vi "Basis VI.vi"() -> ()   [LabVIEW 2013]
uses:
  <vilib>/userdefined/High Color/nirio_resource_hc.ctl
  cRIO_FPGA_COMMUNICATION/TYPES/TYPE Station Index.ctl
  <vilib>/ImagingLab/Kawasaki Robotics Library/typedefs/KwRL-cartesian.ctl
  cRIO_FPGA_COMMUNICATION/GLOBALS/cRIO_FPGA_COMMUNICATION Global.vi
  <vilib>/ImagingLab/Kawasaki Robotics Library/sub/poly/kwrl-motion-move-move_linear(pos).vi
  cRIO_FPGA_COMMUNICATION/cRIO_FPGA_COMMUNICATION.lvlib
  <vilib>/ImagingLab/Kawasaki Robotics Library/KawasakiRoboticsLibrary.lvlib
panel:
  in  "STOP":bool
  in  "WIEDERANFAHRT":bool
  in  "HALT":bool
  in  "START":bool
  in  "demontage oder ausschuss":bool
  in  "Zylinder Festhalten":bool
  in  "Zylinder Bolzen":bool
  in  "value 2":bool
  in  "value":bool
  in  "position 2":T1 {"S" format="%.4g"; "T" format="%.4g"; "A" format="%.4g"; "O" format="%.4g"; "Z" format="%.4g"; "Y" format="%.4g"; "X" format="%.4g"}
  out "MA":bool
  out "Zählerwert 2":u16
  in  "gewünschter Zählerwert 2":u16
  out "Rucksetzen":bool
  in  "Fahr":bool
  in  "Schleichfahrt":bool
  in  "LF":bool
  in  "RF":bool
  out "Impulsgeber":bool
  out "RA":bool
  out "LA":bool
  in  "Band/Station Index (Position im Prozess)":T2
  out "Station":bool[](array[boolean])
  out "Band":bool[](array[boolean])
  in  "Station":bool[](array[boolean])=[FALSE, FALSE, FALSE, FALSE, FALSE, FALSE, FALSE, FALSE]
  in  "Band":bool[](array[boolean])=[FALSE, FALSE, FALSE, FALSE, FALSE, FALSE, FALSE, FALSE]
  in  "Ressourcenname":T3 caption="RIO Device"
  in  "Stopp":bool
  # "Basis VI für allgemeine Stationen"
  # "Senden"
  # "Empfangen"
  # "0      1      2     3     4     5     6     7"
  # "0      1      2     3     4     5     6     7"
  # "Empfangen"
  # "Senden"
  # "0      1      2     3     4     5     6     7"
  # "0      1      2     3     4     5     6     7"
  # "Sensoren"
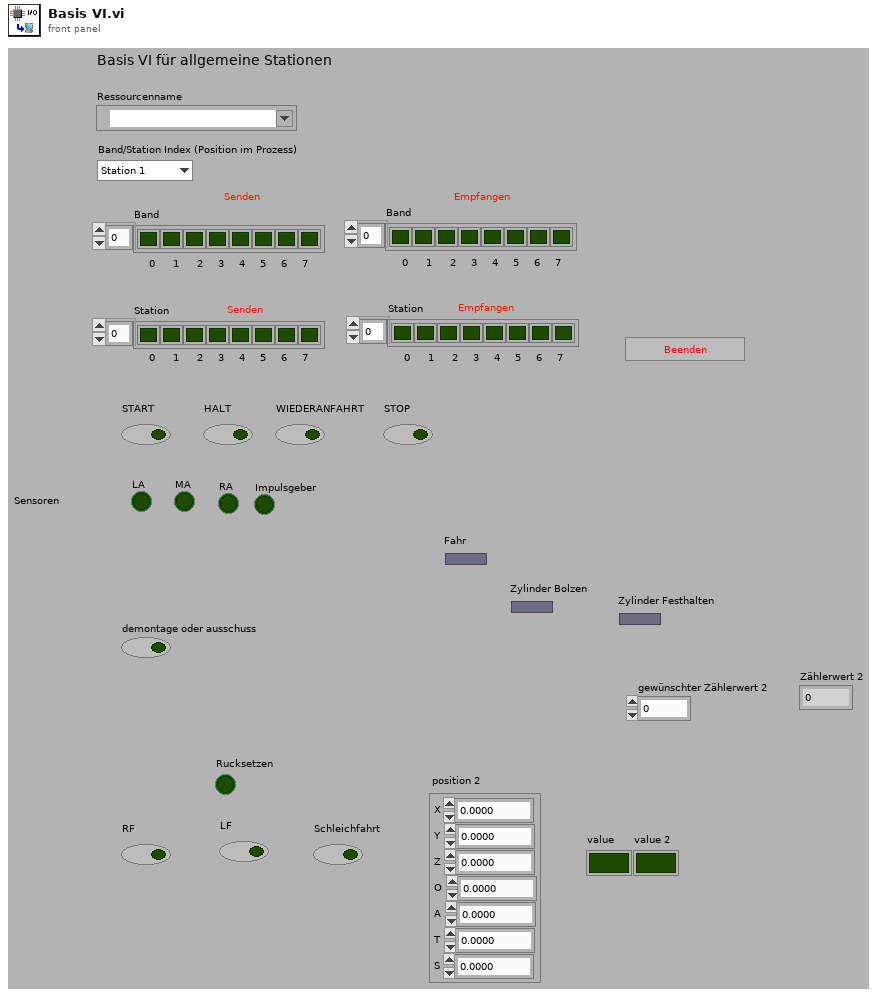
[diagram p1: front panel]
types:
  T1 = typedef "KawasakiRoboticsLibrary.lvlib/kwrl-cartesian.ctl" = cluster{"X":dbl, "Y":dbl, "Z":dbl, "O":dbl, "A":dbl, "T":dbl, "S":dbl}
  T2 = typedef "cRIO_FPGA_COMMUNICATION.lvlib/TYPE Station Index.ctl" = enum16{"Station 1", "Station 2", "Station 3", "Station 4", "Station 5", "Station 6", "Station 7", "Station 8", "Station 9", "Station 10", "Station 11", "Station 12", "Station 13", "Station 14", "Station 15", "Station 16", "Station 17", "Station 18", "Station 19", "Station 20"}
  T3 = typedef "nirio_resource_hc.ctl" = tag
  T4 = typedef "KawasakiRoboticsLibrary.lvlib/KwRL-cartesian.ctl" = cluster{"X":dbl, "Y":dbl, "Z":dbl, "O":dbl, "A":dbl, "T":dbl, "S":dbl}
  T5 = enum16{"Bereit", "Linksfahrt", "Rechtsfahrt 1", "Rechts- und Schleichfahrt", "Stop", "abholen", "demontagepos", "ausschuss", "deckel", "bolzen", "grundkorper", "rechtsfahrt2", "ende"}
  T6 = typedef "TYPE Zählerkonfiguration.ctl" = cluster{"Station/Band":enum16{"Station", "Band"}, "Bitstelle":enum16{"Bit 0", "Bit 1", "Bit 2", "Bit 3", "Bit 4", "Bit 5", "Bit 6", "Bit 7"}, "Zählrichtung":enum16{"Hochzählen", "Runterzählen"}}
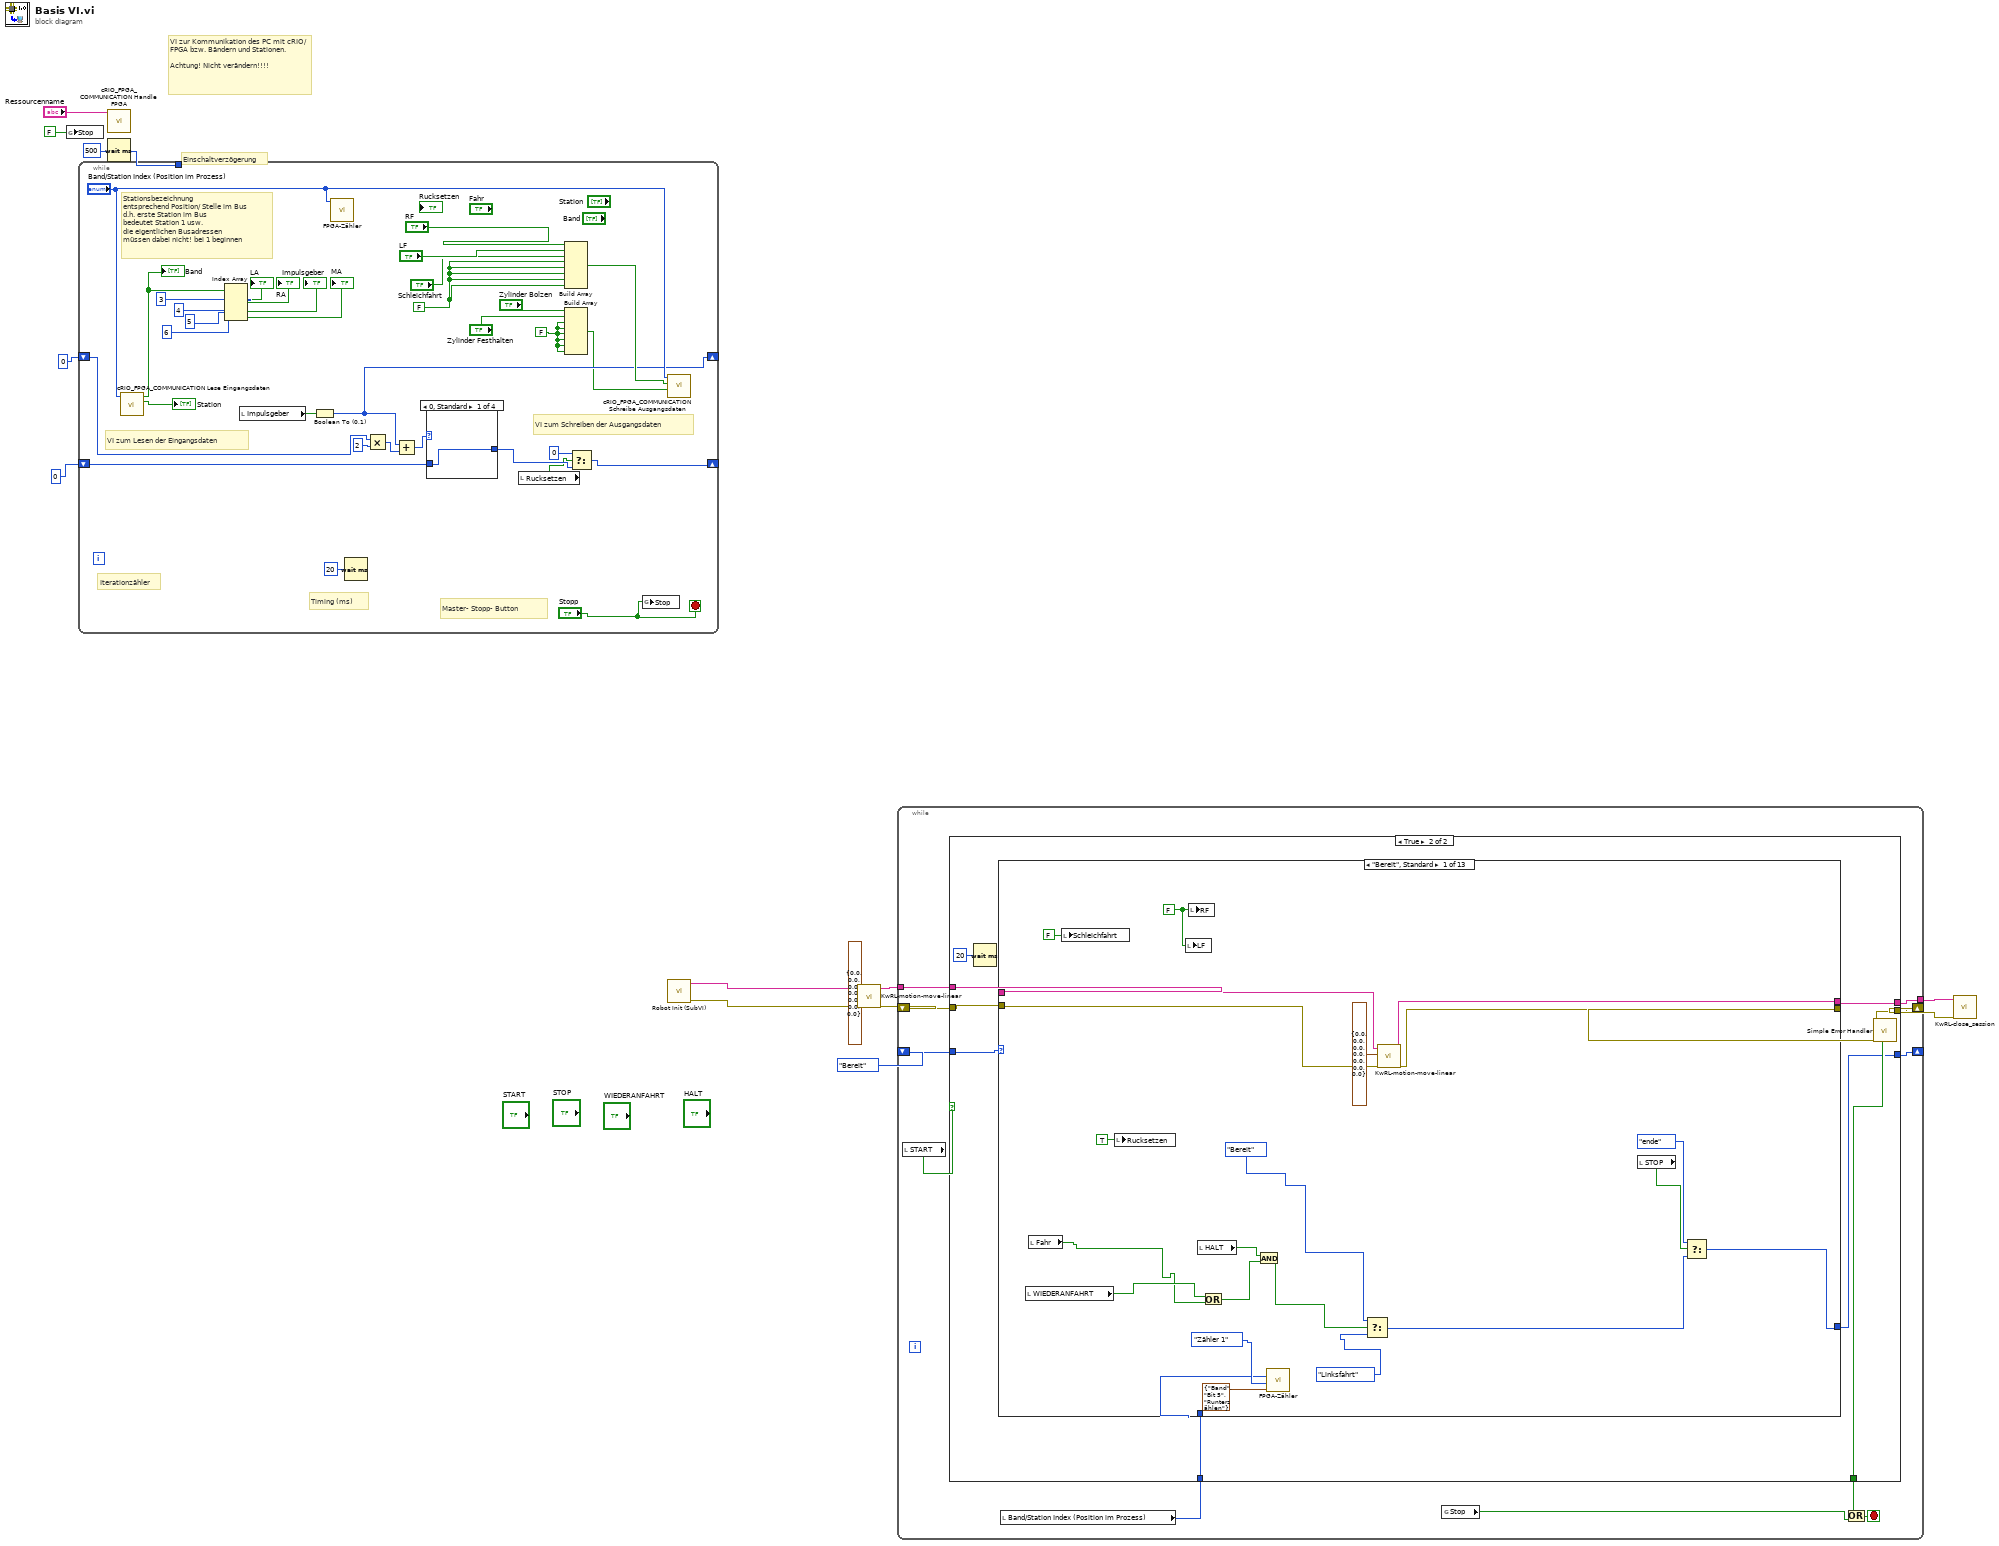
[diagram p0: block diagram]
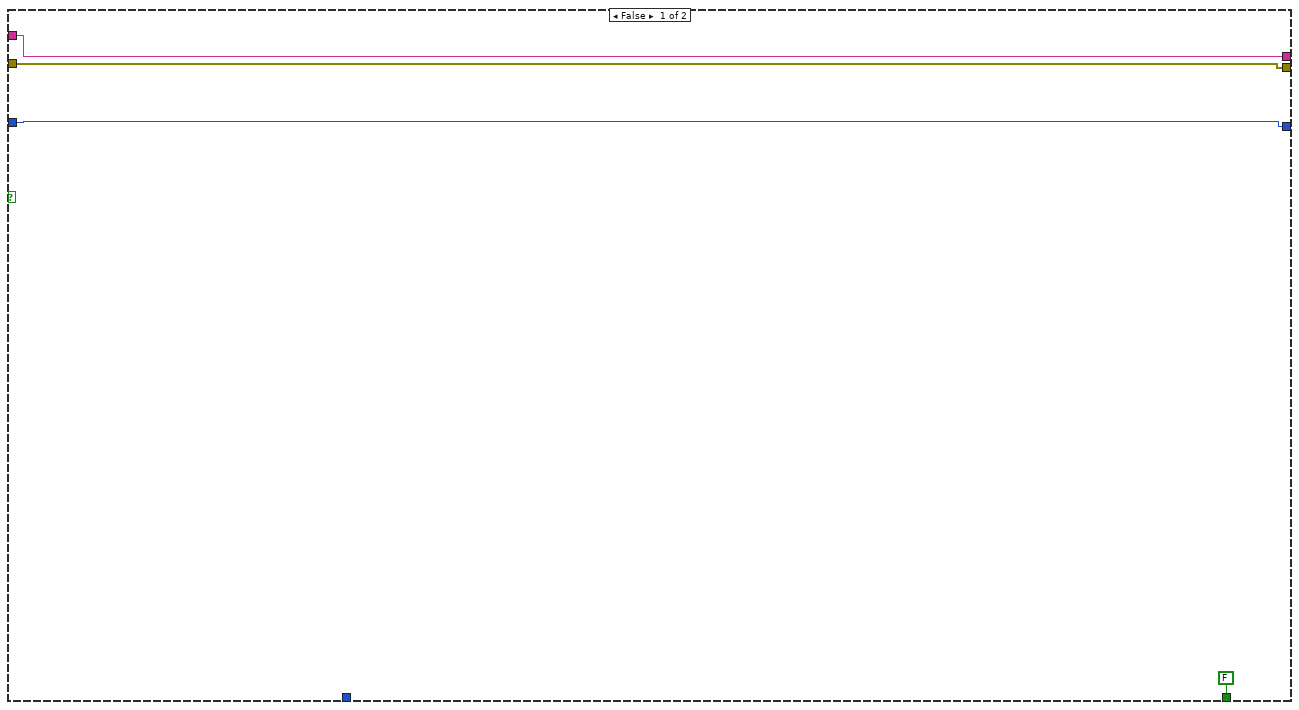
[diagram p2: hidden frame]
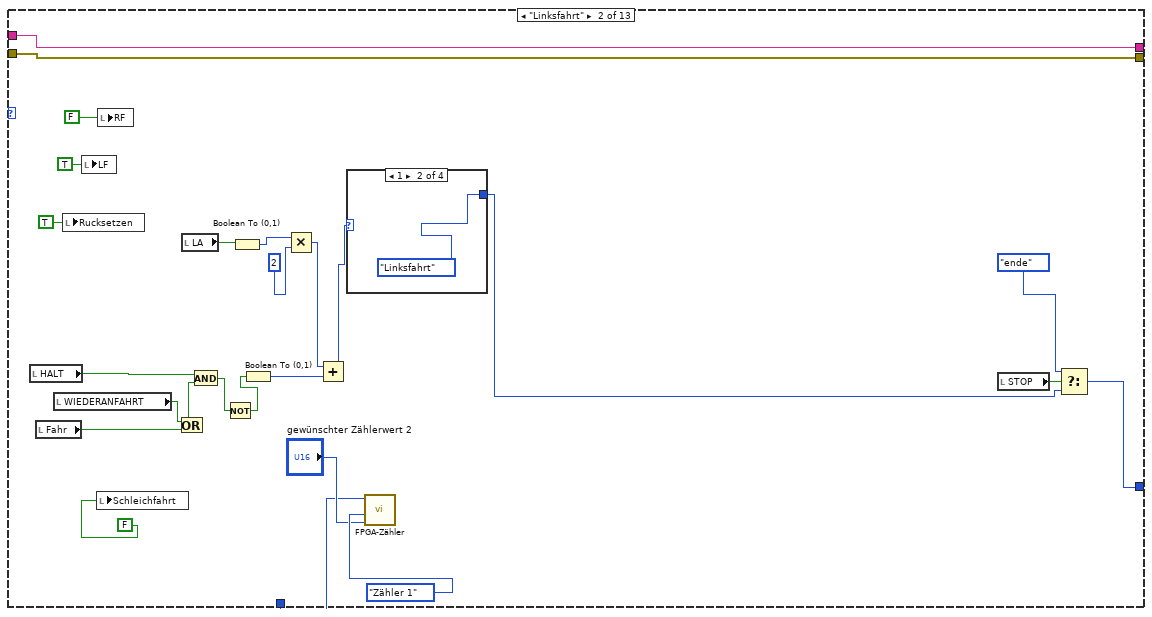
[diagram p3: hidden frame]
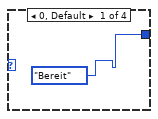
[diagram p4: hidden frame]
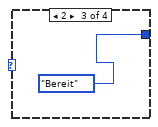
[diagram p5: hidden frame]
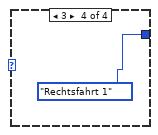
[diagram p6: hidden frame]
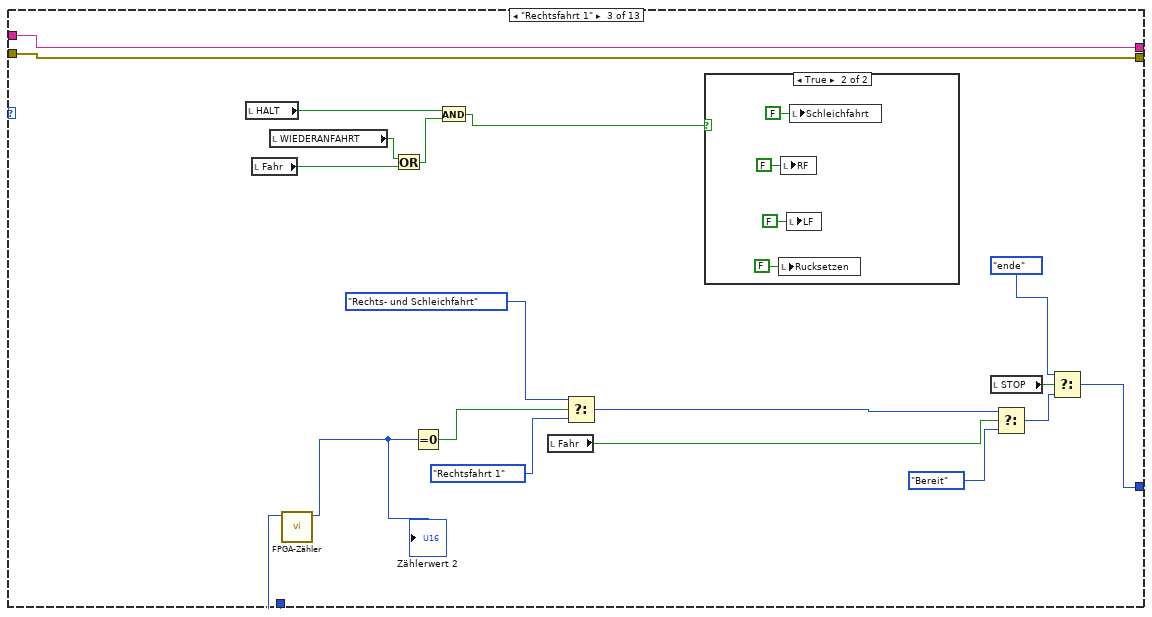
[diagram p7: hidden frame]
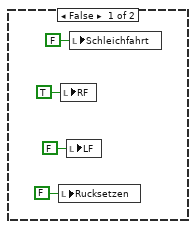
[diagram p8: hidden frame]
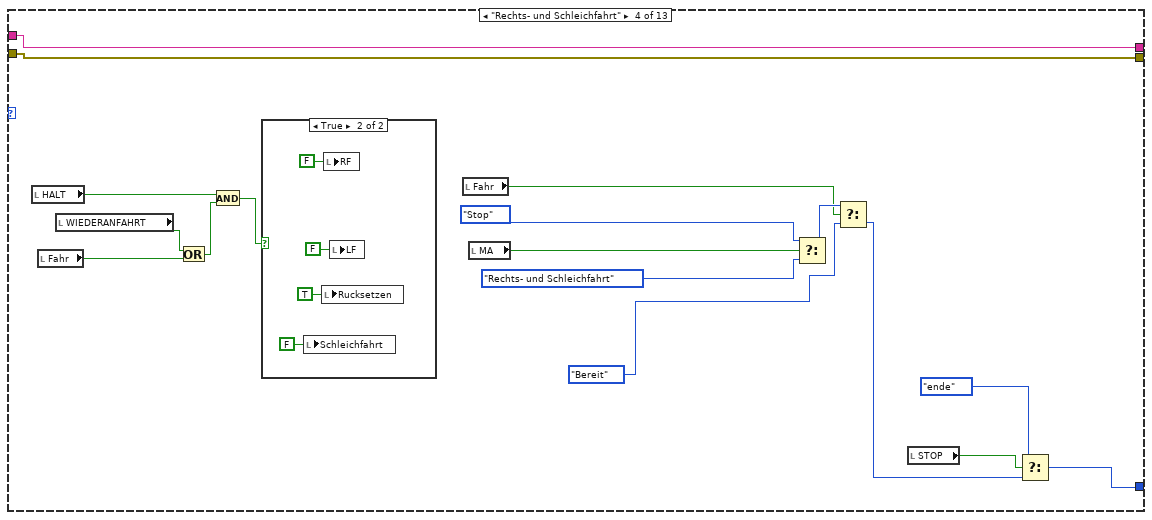
[diagram p9: hidden frame]
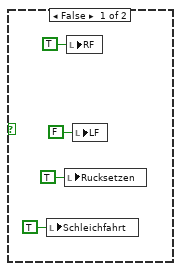
[diagram p10: hidden frame]
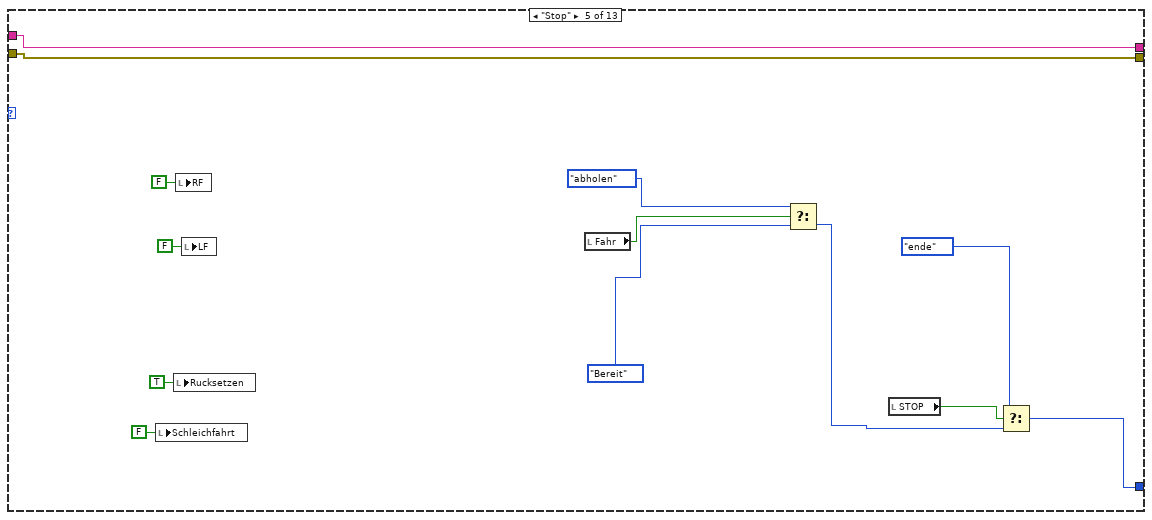
[diagram p11: hidden frame]
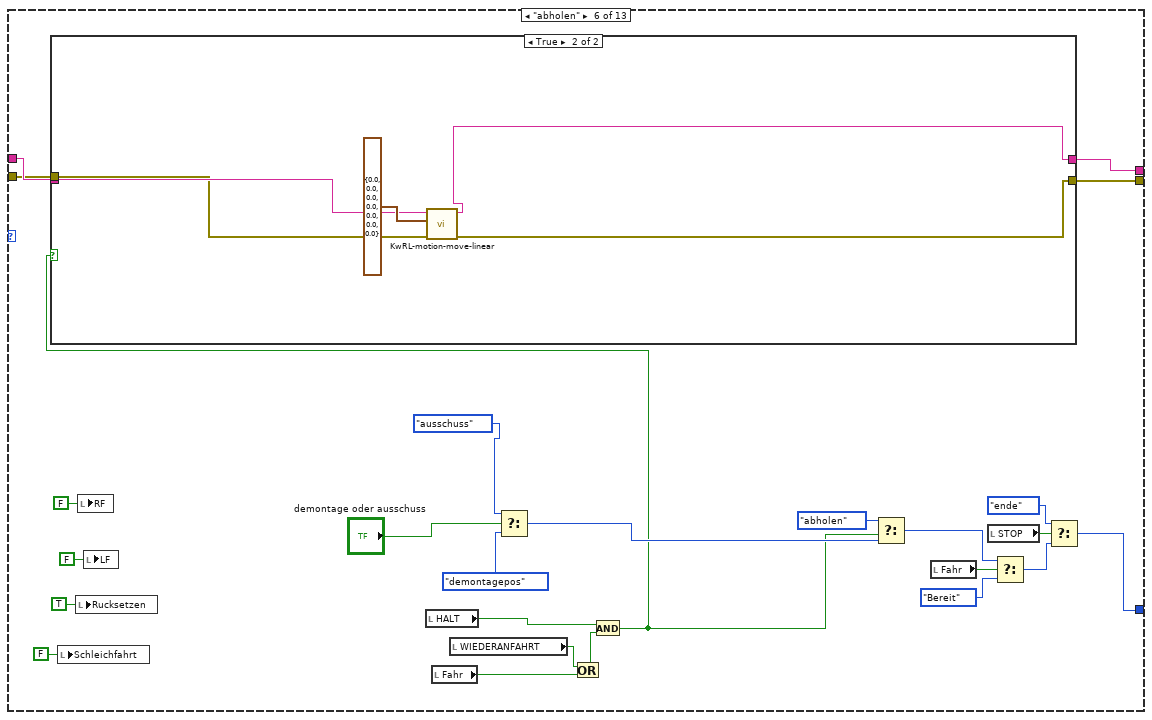
[diagram p12: hidden frame]
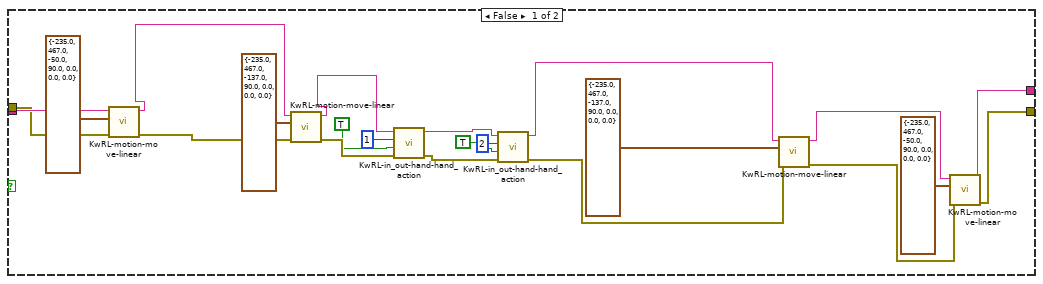
[diagram p13: hidden frame]
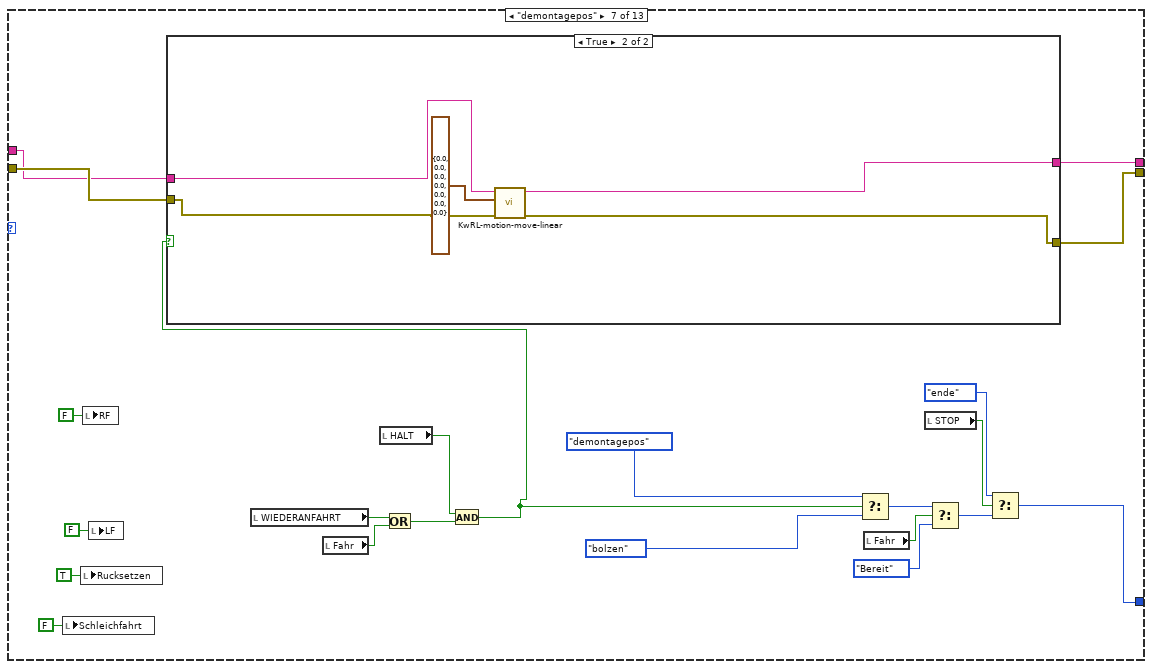
[diagram p14: hidden frame]
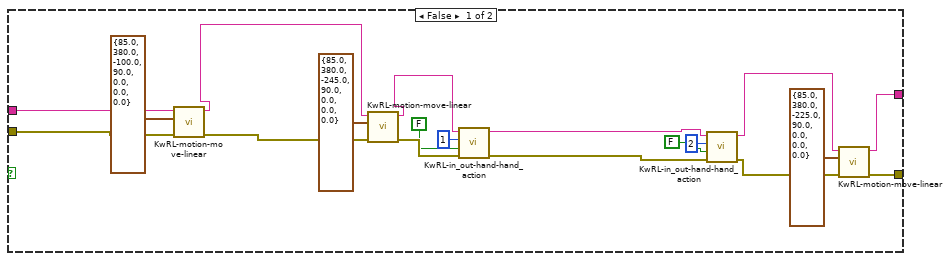
[diagram p15: hidden frame]
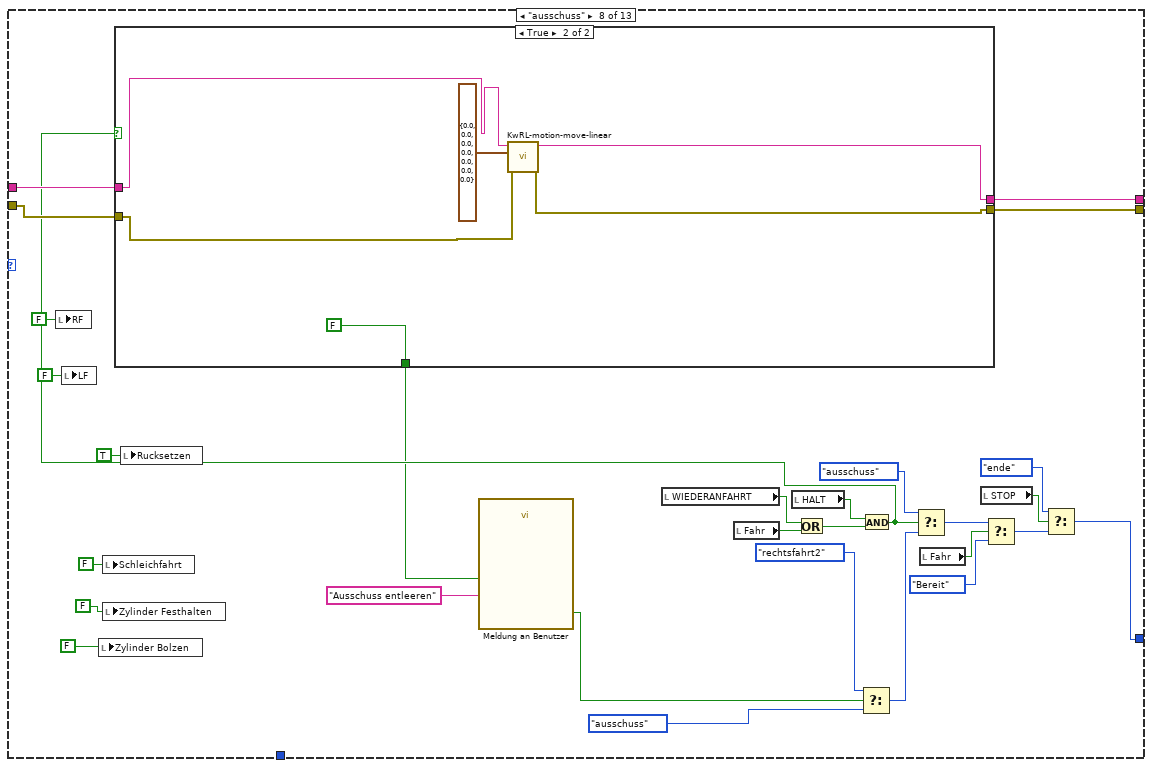
[diagram p16: hidden frame]
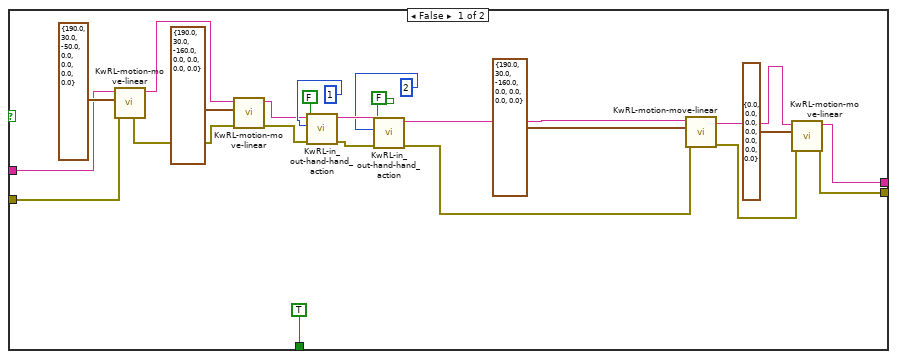
[diagram p17: hidden frame]
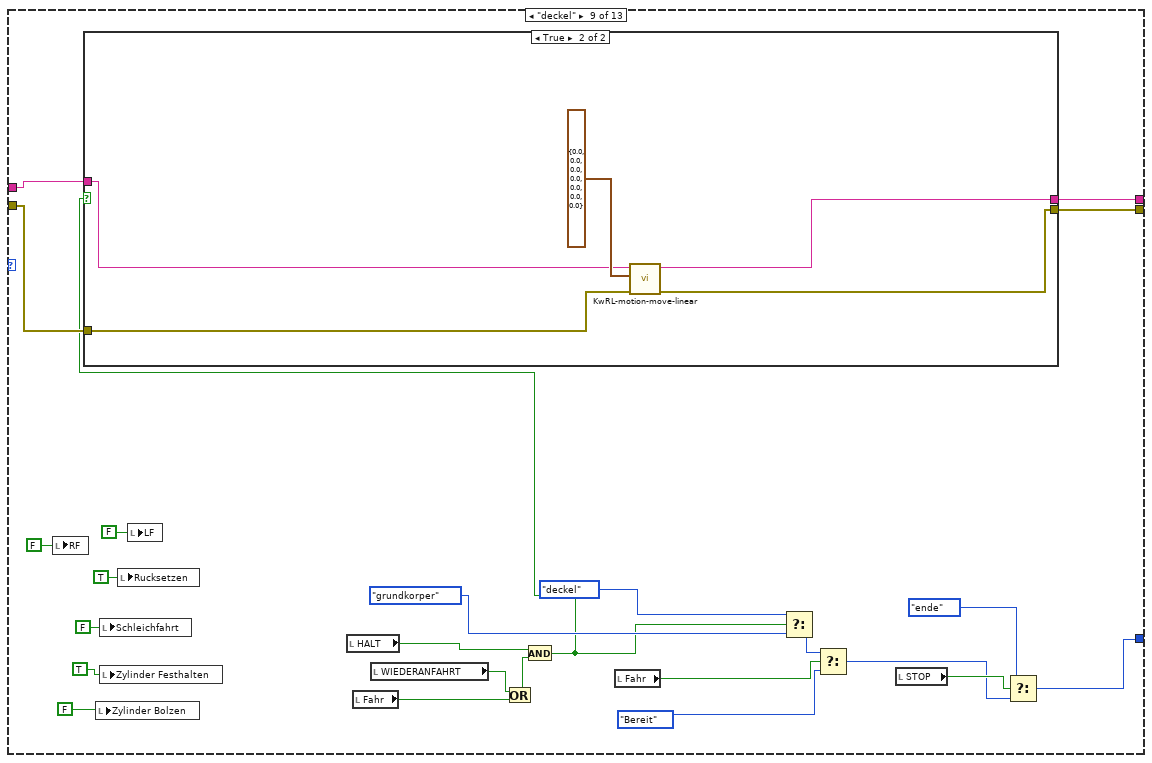
[diagram p18: hidden frame]
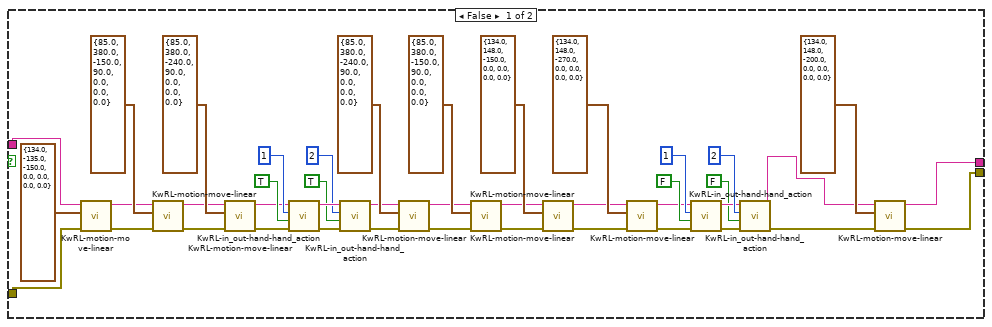
[diagram p19: hidden frame]
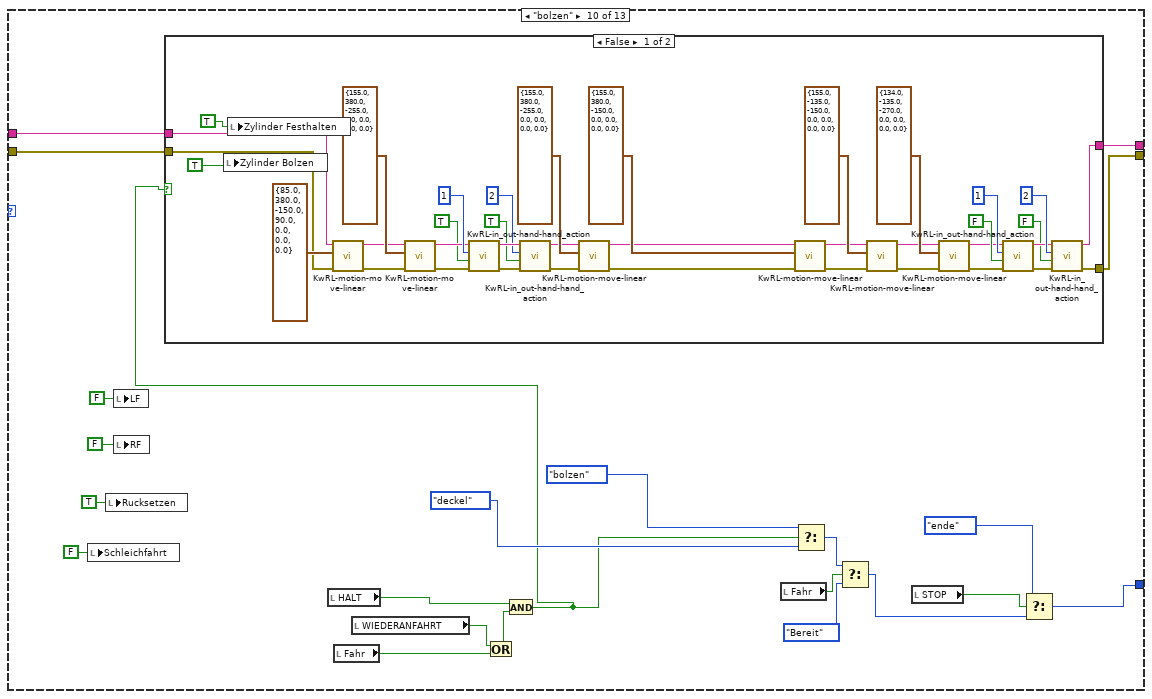
[diagram p20: hidden frame]
diagram:
  # "Einschaltverzögerung"
  # "VI zur Kommunikation des PC mit cRIO/FPGA bzw. Bändern und Stationen. \n\nAchtung! Nicht verändern!!!!"
  n1 = global write "cRIO_FPGA_COMMUNICATION Global.vi" "Stop"(FALSE) -> ()
  n2 = call "cRIO_FPGA_COMMUNICATION Handle FPGA.vi"("Ressourcenname"="Ressourcenname") -> ()  [unwired: 10 in, 1 out]
  n3 = Wait (ms)(milliseconds to wait=u32 500 ("Zu wartende ms")) -> (millisecond timer value=w12:u32)
  n4 = while {
    tunnel: w12 -> [_]
    shift-right: [w31] -> _
    shift-left: i16 0 -> [w33]
    shift-right: [w26] -> _
    shift-left: i16 0 -> [w29]
    stop <- "Stopp" stop-if-true
    w15 = FALSE ("Element")
    w37 = FALSE ("Element")
    # "Timing (ms)"
    # "Iterationzähler"
    # "Stationsbezeichnung\nentsprechend Position/ Stelle im Bus\nd.h. erste Station im Bus\nbedeutet Station 1 usw.\ndie eigentlichen Busadressen \nmüssen dabei nicht! bei 1 beginnen"
    # "Master- Stopp- Button"
    # "VI zum Lesen der Eingangsdaten"
    # "VI zum Schreiben der Ausgangsdaten"
    n5 = call "cRIO_FPGA_COMMUNICATION Lese Eingangsdaten.vi"("Station Index"="Band/Station Index (Position im Prozess)") -> ("Station"=→"Station":bool[], "Band"=w20:bool[])  [unwired: 8 in, 1 out]
    "Band" <- w20
    n6 = Index Array(array=w20, index #1=3 ("Index"), index #2=4 ("Index"), index #3=5 ("Index"), index #4=6 ("Index")) -> (element #1=→"LA":bool, element #2=→"RA":bool, element #3=→"Impulsgeber":bool, element #4=→"MA":bool)
    n7 = local read "Impulsgeber"() -> (w35:bool)
    n8 = Boolean To (0,1)(Boolean=w35) -> (0, 1=w31:i16)
    n9 = call-poly "FPGA-Zähler.vi"("Band/Station Index"="Band/Station Index (Position im Prozess)") -> ()  [unwired: 8 in, 3 out]
    n10 = Wait (ms)(milliseconds to wait=u32 20 ("Zu wartende ms")) -> ()  [unwired: 1 out]
    n11 = Multiply(x=w33, y=i16 2) -> (x*y=w32:i16)
    n12 = Add(x=w31, y=w32) -> (x+y=w30:i16)
    n13 = case shown="0, Standard" w30 {
      tunnel: w29 -> [w48 w50 w51 w52]
      tunnel: [w48 w49 w51 w52] -> w28
      frame 0, Default {
      }
      frame 1 {
        n14 = Increment(x=w50) -> (x+1=w49:i16)
      }
      frame 2 {
      }
      frame 3 {
      }
    }
    n15 = local read "Rucksetzen"() -> (w25:bool)
    n16 = Build Array("RF", "LF", "Schleichfahrt", w37, w37, w37, w37, w37) -> (w36:bool[])
    n17 = Build Array("Zylinder Bolzen", "Zylinder Festhalten", w15, w15, w15, w15, w15, w15) -> (w18:bool[])
    n18 = Select(t=i16 0, s=w25, f=w28) -> (s? t:f=w26:i16)
    n19 = global write "cRIO_FPGA_COMMUNICATION Global.vi" "Stop"("Stopp") -> ()
    n20 = call "cRIO_FPGA_COMMUNICATION Schreibe Ausgangsdaten.vi"("Station"=w18, "Band"=w36, "Station Index"="Band/Station Index (Position im Prozess)") -> ()  [unwired: 8 in, 1 out]
  }
  n21 = call "Robot Init (SubVI).vi"() -> ("Fehler (Ausgang)"=w7:errorcluster, "robot session*"=w8:string)  [unwired: 10 in]
  n22 = call-poly <vilib>:"KwRL-motion-move-linear.vi"("error in"=w7, "position"=T4 {"X"=0.0, "Y"=0.0, "Z"=0.0, "O"=0.0, "A"=0.0, "T"=0.0, "S"=0.0}, "robot session"=w8) -> ("error out"=w3:errorcluster, "robot session*"=w4:string)  [unwired: 7 in]
  n23 = while {
    tunnel: [w63] -> w5
    tunnel: w4 -> [w62]
    shift-right: [w60] -> w2
    shift-left: w3 -> [w61]
    shift-right: [w54] -> _
    shift-left: T5."Bereit" -> [w55]
    stop <- w56 stop-if-true
    n24 = local read "START"() -> (w53:bool)
    n25 = local read "Band/Station Index (Position im Prozess)"() -> (w59:T2)
    n26 = case shown="True" w53 {
      tunnel: [w65 w76] -> w63
      tunnel: w62 -> [w65 w75]
      tunnel: w61 -> [w66 w73]
      tunnel: [w66 w72] -> w60
      tunnel: w59 -> [_ w71]
      tunnel: [FALSE ("error?") w70] -> w57
      tunnel: w55 -> [w67 w69]
      tunnel: [w67 w68] -> w54
      frame False {
      }
      frame True {
        n27 = Wait (ms)(milliseconds to wait=u32 20 ("Zu wartende ms")) -> ()  [unwired: 1 out]
        n28 = case shown="\"Bereit\", Standard" w69 {
          tunnel: [w96 w112 w142 w168 w188 w211 w249 w310 w365 w435 w502 w575 w594] -> w76
          tunnel: w75 -> [w97 w112 w142 w168 w188 w214 w262 w314 w367 w442 w504 w575 w604]
          tunnel: [w98 w113 w143 w169 w189 w212 w248 w309 w364 w436 w503 w574 w595] -> w74
          tunnel: w73 -> [w99 w113 w143 w169 w189 w213 w263 w313 w368 w441 w505 w574 w607]
          tunnel: [w85 w109 w134 w161 w181 w202 w256 w304 w358 w429 w496 w564 T5."ende"] -> w68
          tunnel: w71 -> [w90 w122 w147 _ _ _ _ _ _ _ _ _ _]
          frame "Bereit", Default {
            w94 = FALSE ("RF")
            n29 = local read "WIEDERANFAHRT"() -> (w81:bool)
            n30 = local read "Fahr"() -> (w80:bool)
            n31 = local write "Schleichfahrt"(FALSE ("Schleichfahrt")) -> ()
            n32 = local write "Rucksetzen"(TRUE ("Rucksetzen")) -> ()
            n33 = local write "LF"(w94) -> ()
            n34 = local write "RF"(w94) -> ()
            n35 = local read "HALT"() -> (w82:bool)
            n36 = Or(x=w81, y=w80) -> (x .or. y?=w79:bool)
            n37 = And(x=w82, y=w79) -> (x .and. y?=w84:bool)
            n38 = call-poly "FPGA-Zähler.vi"("Konfiguration"=T6 {"Station/Band"=enum."Band", "Bitstelle"=enum."Bit 5", "Zählrichtung"=enum."Runterzählen"}, "Zähler"=enum16{"Zähler 1", "Zähler 2", "Zähler 3"}."Zähler 1", "Band/Station Index"=w90) -> ()  [unwired: 9 in]
            n39 = Select(t=T5."Bereit", s=w84, f=T5."Linksfahrt") -> (s? t:f=w83:T5)
            n40 = call-poly <vilib>:"KwRL-motion-move-linear.vi"("error in"=w99, "position"=T4 {"X"=0.0, "Y"=0.0, "Z"=0.0, "O"=0.0, "A"=0.0, "T"=0.0, "S"=0.0}, "robot session"=w97) -> ("error out"=w98:errorcluster, "robot session*"=w96:string)  [unwired: 7 in]
            n41 = local read "STOP"() -> (w87:bool)
            n42 = Select(t=T5."ende", s=w87, f=w83) -> (s? t:f=w85:T5)
          }
          frame "Linksfahrt" {
            n43 = local read "HALT"() -> (w107:bool)
            n44 = local read "Fahr"() -> (w105:bool)
            n45 = local read "WIEDERANFAHRT"() -> (w106:bool)
            n46 = local write "Rucksetzen"(TRUE ("Rucksetzen")) -> ()
            n47 = local write "LF"(TRUE ("LF")) -> ()
            n48 = local write "Schleichfahrt"(FALSE ("Schleichfahrt")) -> ()
            n49 = local write "RF"(FALSE ("RF")) -> ()
            n50 = Or(x=w106, y=w105) -> (x .or. y?=w104:bool)
            n51 = local read "LA"() -> (w114:bool)
            n52 = And(x=w107, y=w104) -> (x .and. y?=w102:bool)
            n53 = Not(x=w102) -> (.not. x?=w101:bool)
            n54 = Boolean To (0,1)(Boolean=w114) -> (0, 1=w115:i16)
            n55 = Boolean To (0,1)(Boolean=w101) -> (0, 1=w118:i16)
            n56 = Multiply(x=w115, y=i16 2) -> (x*y=w117:i16)
            n57 = Add(x=w117, y=w118) -> (x+y=w119:i16)
            n58 = case shown="1" w119 {
              tunnel: [T5."Bereit" T5."Linksfahrt" T5."Bereit" T5."Rechtsfahrt 1"] -> w103
              frame 0, Default {
              }
              frame 1 {
              }
              frame 2 {
              }
              frame 3 {
              }
            }
            n59 = call-poly "FPGA-Zähler.vi"("gewünschter Zählerwert"="gewünschter Zählerwert 2", "Zähler"=enum16{"Zähler 1", "Zähler 2", "Zähler 3"}."Zähler 1", "Band/Station Index"=w122) -> ()  [unwired: 9 in]
            n60 = local read "STOP"() -> (w111:bool)
            n61 = Select(t=T5."ende", s=w111, f=w103) -> (s? t:f=w109:T5)
          }
          frame "Rechtsfahrt 1" {
            n62 = local read "HALT"() -> (w133:bool)
            n63 = local read "Fahr"() -> (w131:bool)
            n64 = local read "WIEDERANFAHRT"() -> (w132:bool)
            n65 = call-poly "FPGA-Zähler.vi"("Band/Station Index"=w147) -> ("Zählerwert 1"=w141:u16)  [unwired: 8 in, 2 out]
            "Zählerwert 2" <- w141
            n66 = Or(x=w132, y=w131) -> (x .or. y?=w130:bool)
            n67 = Equal To 0?(x=w141) -> (x = 0?=w146:bool)
            n68 = And(x=w133, y=w130) -> (x .and. y?=w129:bool)
            n69 = local read "Fahr"() -> (w144:bool)
            n70 = Select(t=T5."Rechts- und Schleichfahrt", s=w146, f=T5."Rechtsfahrt 1") -> (s? t:f=w145:T5)
            n71 = case shown="True" w129 {
              frame False {
                n72 = local write "Rucksetzen"(FALSE ("Rucksetzen")) -> ()
                n73 = local write "RF"(TRUE ("RF")) -> ()
                n74 = local write "LF"(FALSE ("LF")) -> ()
                n75 = local write "Schleichfahrt"(FALSE ("Schleichfahrt")) -> ()
              }
              frame True {
                n76 = local write "Rucksetzen"(FALSE ("Rucksetzen")) -> ()
                n77 = local write "RF"(FALSE ("RF")) -> ()
                n78 = local write "LF"(FALSE ("LF")) -> ()
                n79 = local write "Schleichfahrt"(FALSE ("Schleichfahrt")) -> ()
              }
            }
            n80 = local read "STOP"() -> (w137:bool)
            n81 = Select(t=w145, s=w144, f=T5."Bereit") -> (s? t:f=w135:T5)
            n82 = Select(t=T5."ende", s=w137, f=w135) -> (s? t:f=w134:T5)
          }
          frame "Rechts- und Schleichfahrt" {
            n83 = local read "HALT"() -> (w160:bool)
            n84 = local read "Fahr"() -> (w158:bool)
            n85 = local read "WIEDERANFAHRT"() -> (w159:bool)
            n86 = Or(x=w159, y=w158) -> (x .or. y?=w157:bool)
            n87 = And(x=w160, y=w157) -> (x .and. y?=w156:bool)
            n88 = case shown="True" w156 {
              frame False {
                n89 = local write "Schleichfahrt"(TRUE ("Schleichfahrt")) -> ()
                n90 = local write "Rucksetzen"(TRUE ("Rucksetzen")) -> ()
                n91 = local write "RF"(TRUE ("RF")) -> ()
                n92 = local write "LF"(FALSE ("LF")) -> ()
              }
              frame True {
                n93 = local write "Schleichfahrt"(FALSE ("Schleichfahrt")) -> ()
                n94 = local write "Rucksetzen"(TRUE ("Rucksetzen")) -> ()
                n95 = local write "RF"(FALSE ("RF")) -> ()
                n96 = local write "LF"(FALSE ("LF")) -> ()
              }
            }
            n97 = local read "Fahr"() -> (w171:bool)
            n98 = local read "MA"() -> (w170:bool)
            n99 = Select(t=T5."Stop", s=w170, f=T5."Rechts- und Schleichfahrt") -> (s? t:f=w172:T5)
            n100 = Select(t=w172, s=w171, f=T5."Bereit") -> (s? t:f=w162:T5)
            n101 = local read "STOP"() -> (w164:bool)
            n102 = Select(t=T5."ende", s=w164, f=w162) -> (s? t:f=w161:T5)
          }
          frame "Stop" {
            n103 = local write "Schleichfahrt"(FALSE ("Schleichfahrt")) -> ()
            n104 = local write "Rucksetzen"(TRUE ("Rucksetzen")) -> ()
            n105 = local write "RF"(FALSE ("RF")) -> ()
            n106 = local write "LF"(FALSE ("LF")) -> ()
            n107 = local read "Fahr"() -> (w187:bool)
            n108 = Select(t=T5."abholen", s=w187, f=T5."Bereit") -> (s? t:f=w182:T5)
            n109 = local read "STOP"() -> (w184:bool)
            n110 = Select(t=T5."ende", s=w184, f=w182) -> (s? t:f=w181:T5)
          }
          frame "abholen" {
            n111 = local write "Schleichfahrt"(FALSE ("Schleichfahrt")) -> ()
            n112 = local write "Rucksetzen"(TRUE ("Rucksetzen")) -> ()
            n113 = local write "RF"(FALSE ("RF")) -> ()
            n114 = local write "LF"(FALSE ("LF")) -> ()
            n115 = local read "HALT"() -> (w198:bool)
            n116 = local read "Fahr"() -> (w200:bool)
            n117 = local read "WIEDERANFAHRT"() -> (w199:bool)
            n118 = Select(t=T5."ausschuss", s="demontage oder ausschuss", f=T5."demontagepos") -> (s? t:f=w196:T5)
            n119 = Or(x=w199, y=w200) -> (x .or. y?=w201:bool)
            n120 = And(x=w198, y=w201) -> (x .and. y?=w194:bool)
            n121 = case shown="True" w194 {
              tunnel: w214 -> [w240 w244]
              tunnel: w213 -> [w239 w243]
              tunnel: [w225 w241] -> w212
              tunnel: [w224 w242] -> w211
              frame False {
                n122 = call-poly <vilib>:"KwRL-motion-move-linear.vi"("error in"=w239, "position"=T4 {"X"=-235.0, "Y"=467.0, "Z"=-50.0, "O"=90.0, "A"=0.0, "T"=0.0, "S"=0.0}, "robot session"=w240) -> ("error out"=w236:errorcluster, "robot session*"=w237:string)  [unwired: 7 in]
                n123 = call-poly <vilib>:"KwRL-motion-move-linear.vi"("error in"=w236, "position"=T4 {"X"=-235.0, "Y"=467.0, "Z"=-137.0, "O"=90.0, "A"=0.0, "T"=0.0, "S"=0.0}, "robot session"=w237) -> ("error out"=w231:errorcluster, "robot session*"=w232:string)  [unwired: 7 in]
                n124 = call <vilib>:"KwRL-in_out-hand-hand_action.vi"("error in"=w231, "value"=TRUE, "clamp"=i16 1, "robot session"=w232) -> ("error out"=w230:errorcluster, "robot session*"=w229:string)  [unwired: 6 in]
                n125 = call <vilib>:"KwRL-in_out-hand-hand_action.vi"("error in"=w230, "value"=TRUE, "clamp"=i16 2, "robot session"=w229) -> ("error out"=w219:errorcluster, "robot session*"=w222:string)  [unwired: 6 in]
                n126 = call-poly <vilib>:"KwRL-motion-move-linear.vi"("error in"=w219, "position"=T4 {"X"=-235.0, "Y"=467.0, "Z"=-137.0, "O"=90.0, "A"=0.0, "T"=0.0, "S"=0.0}, "robot session"=w222) -> ("error out"=w221:errorcluster, "robot session*"=w220:string)  [unwired: 7 in]
                n127 = call-poly <vilib>:"KwRL-motion-move-linear.vi"("error in"=w221, "position"=T4 {"X"=-235.0, "Y"=467.0, "Z"=-50.0, "O"=90.0, "A"=0.0, "T"=0.0, "S"=0.0}, "robot session"=w220) -> ("error out"=w225:errorcluster, "robot session*"=w224:string)  [unwired: 7 in]
              }
              frame True {
                n128 = call-poly <vilib>:"KwRL-motion-move-linear.vi"("error in"=w243, "position"=T4 {"X"=0.0, "Y"=0.0, "Z"=0.0, "O"=0.0, "A"=0.0, "T"=0.0, "S"=0.0}, "robot session"=w244) -> ("error out"=w241:errorcluster, "robot session*"=w242:string)  [unwired: 7 in]
              }
            }
            n129 = Select(t=T5."abholen", s=w194, f=w196) -> (s? t:f=w197:T5)
            n130 = local read "Fahr"() -> (w210:bool)
            n131 = local read "STOP"() -> (w205:bool)
            n132 = Select(t=w197, s=w210, f=T5."Bereit") -> (s? t:f=w203:T5)
            n133 = Select(t=T5."ende", s=w205, f=w203) -> (s? t:f=w202:T5)
          }
          frame "demontagepos" {
            n134 = local write "Schleichfahrt"(FALSE ("Schleichfahrt")) -> ()
            n135 = local write "Rucksetzen"(TRUE ("Rucksetzen")) -> ()
            n136 = local write "RF"(FALSE ("RF")) -> ()
            n137 = local write "LF"(FALSE ("LF")) -> ()
            n138 = local read "WIEDERANFAHRT"() -> (w253:bool)
            n139 = local read "Fahr"() -> (w254:bool)
            n140 = local read "HALT"() -> (w252:bool)
            n141 = Or(x=w253, y=w254) -> (x .or. y?=w255:bool)
            n142 = And(x=w252, y=w255) -> (x .and. y?=w246:bool)
            n143 = case shown="True" w246 {
              tunnel: w263 -> [w271 w290]
              tunnel: w262 -> [w270 w287]
              tunnel: [w269 w289] -> w249
              tunnel: [w268 w288] -> w248
              frame False {
                n144 = call-poly <vilib>:"KwRL-motion-move-linear.vi"("error in"=w271, "position"=T4 {"X"=85.0, "Y"=380.0, "Z"=-100.0, "O"=90.0, "A"=0.0, "T"=0.0, "S"=0.0}, "robot session"=w270) -> ("error out"=w284:errorcluster, "robot session*"=w285:string)  [unwired: 7 in]
                n145 = call-poly <vilib>:"KwRL-motion-move-linear.vi"("error in"=w284, "position"=T4 {"X"=85.0, "Y"=380.0, "Z"=-245.0, "O"=90.0, "A"=0.0, "T"=0.0, "S"=0.0}, "robot session"=w285) -> ("error out"=w279:errorcluster, "robot session*"=w280:string)  [unwired: 7 in]
                n146 = call <vilib>:"KwRL-in_out-hand-hand_action.vi"("error in"=w279, "value"=FALSE, "clamp"=i16 1, "robot session"=w280) -> ("error out"=w278:errorcluster, "robot session*"=w277:string)  [unwired: 6 in]
                n147 = call <vilib>:"KwRL-in_out-hand-hand_action.vi"("error in"=w278, "value"=FALSE, "clamp"=i16 2, "robot session"=w277) -> ("error out"=w273:errorcluster, "robot session*"=w272:string)  [unwired: 6 in]
                n148 = call-poly <vilib>:"KwRL-motion-move-linear.vi"("error in"=w273, "position"=T4 {"X"=85.0, "Y"=380.0, "Z"=-225.0, "O"=90.0, "A"=0.0, "T"=0.0, "S"=0.0}, "robot session"=w272) -> ("error out"=w268:errorcluster, "robot session*"=w269:string)  [unwired: 7 in]
              }
              frame True {
                n149 = call-poly <vilib>:"KwRL-motion-move-linear.vi"("error in"=w290, "position"=T4 {"X"=0.0, "Y"=0.0, "Z"=0.0, "O"=0.0, "A"=0.0, "T"=0.0, "S"=0.0}, "robot session"=w287) -> ("error out"=w288:errorcluster, "robot session*"=w289:string)  [unwired: 7 in]
              }
            }
            n150 = Select(t=T5."demontagepos", s=w246, f=T5."bolzen") -> (s? t:f=w250:T5)
            n151 = local read "Fahr"() -> (w261:bool)
            n152 = local read "STOP"() -> (w259:bool)
            n153 = Select(t=w250, s=w261, f=T5."Bereit") -> (s? t:f=w257:T5)
            n154 = Select(t=T5."ende", s=w259, f=w257) -> (s? t:f=w256:T5)
          }
          frame "ausschuss" {
            n155 = local write "RF"(FALSE ("RF")) -> ()
            n156 = local write "LF"(FALSE ("LF")) -> ()
            n157 = local write "Zylinder Bolzen"(FALSE ("Rucksetzen")) -> ()
            n158 = local write "Schleichfahrt"(FALSE ("Schleichfahrt")) -> ()
            n159 = local write "Zylinder Festhalten"(FALSE ("Rucksetzen")) -> ()
            n160 = local write "Rucksetzen"(TRUE ("Rucksetzen")) -> ()
            n161 = local read "WIEDERANFAHRT"() -> (w300:bool)
            n162 = local read "Fahr"() -> (w301:bool)
            n163 = local read "HALT"() -> (w299:bool)
            n164 = Or(x=w300, y=w301) -> (x .or. y?=w302:bool)
            n165 = And(x=w299, y=w302) -> (x .and. y?=w295:bool)
            n166 = case shown="True" w295 {
              tunnel: w314 -> [w325 w348]
              tunnel: w313 -> [w324 w347]
              tunnel: [w323 w345] -> w310
              tunnel: [w322 w346] -> w309
              tunnel: [TRUE ("Enable") FALSE ("OK")] -> w293
              frame False {
                n167 = call-poly <vilib>:"KwRL-motion-move-linear.vi"("error in"=w324, "position"=T4 {"X"=190.0, "Y"=30.0, "Z"=-50.0, "O"=0.0, "A"=0.0, "T"=0.0, "S"=0.0}, "robot session"=w325) -> ("error out"=w340:errorcluster, "robot session*"=w341:string)  [unwired: 7 in]
                n168 = call-poly <vilib>:"KwRL-motion-move-linear.vi"("error in"=w340, "position"=T4 {"X"=190.0, "Y"=30.0, "Z"=-160.0, "O"=0.0, "A"=0.0, "T"=0.0, "S"=0.0}, "robot session"=w341) -> ("error out"=w326:errorcluster, "robot session*"=w327:string)  [unwired: 7 in]
                n169 = call <vilib>:"KwRL-in_out-hand-hand_action.vi"("error in"=w326, "value"=FALSE, "clamp"=i16 1, "robot session"=w327) -> ("error out"=w338:errorcluster, "robot session*"=w339:string)  [unwired: 6 in]
                n170 = call <vilib>:"KwRL-in_out-hand-hand_action.vi"("error in"=w338, "value"=FALSE, "clamp"=i16 2, "robot session"=w339) -> ("error out"=w329:errorcluster, "robot session*"=w334:string)  [unwired: 6 in]
                n171 = call-poly <vilib>:"KwRL-motion-move-linear.vi"("error in"=w329, "position"=T4 {"X"=190.0, "Y"=30.0, "Z"=-160.0, "O"=0.0, "A"=0.0, "T"=0.0, "S"=0.0}, "robot session"=w334) -> ("error out"=w328:errorcluster, "robot session*"=w330:string)  [unwired: 7 in]
                n172 = call-poly <vilib>:"KwRL-motion-move-linear.vi"("error in"=w328, "position"=T4 {"X"=0.0, "Y"=0.0, "Z"=0.0, "O"=0.0, "A"=0.0, "T"=0.0, "S"=0.0}, "robot session"=w330) -> ("error out"=w322:errorcluster, "robot session*"=w323:string)  [unwired: 7 in]
              }
              frame True {
                n173 = call-poly <vilib>:"KwRL-motion-move-linear.vi"("error in"=w347, "position"=T4 {"X"=0.0, "Y"=0.0, "Z"=0.0, "O"=0.0, "A"=0.0, "T"=0.0, "S"=0.0}, "robot session"=w348) -> ("error out"=w346:errorcluster, "robot session*"=w345:string)  [unwired: 7 in]
              }
            }
            n174 = call "Meldung an Benutzer"("Enable"=w293, "Message"="Ausschuss entleeren") -> ("OK"=w292:bool)  [unwired: 8 in, 1 out]
            n175 = Select(t=T5."rechtsfahrt2", s=w292, f=T5."ausschuss") -> (s? t:f=w297:T5)
            n176 = Select(t=T5."ausschuss", s=w295, f=w297) -> (s? t:f=w298:T5)
            n177 = local read "Fahr"() -> (w312:bool)
            n178 = local read "STOP"() -> (w306:bool)
            n179 = Select(t=w298, s=w312, f=T5."Bereit") -> (s? t:f=w303:T5)
            n180 = Select(t=T5."ende", s=w306, f=w303) -> (s? t:f=w304:T5)
          }
          frame "deckel" {
            n181 = local write "RF"(FALSE ("RF")) -> ()
            n182 = local write "Zylinder Bolzen"(FALSE ("Rucksetzen")) -> ()
            n183 = local write "Schleichfahrt"(FALSE ("Schleichfahrt")) -> ()
            n184 = local write "Zylinder Festhalten"(TRUE ("Rucksetzen")) -> ()
            n185 = local write "Rucksetzen"(TRUE ("Rucksetzen")) -> ()
            n186 = local write "LF"(FALSE ("LF")) -> ()
            n187 = local read "HALT"() -> (w355:bool)
            n188 = local read "Fahr"() -> (w351:bool)
            n189 = local read "WIEDERANFAHRT"() -> (w356:bool)
            n190 = Or(x=w356, y=w351) -> (x .or. y?=w357:bool)
            n191 = And(x=w355, y=w357) -> (x .and. y?=w350:bool)
            n192 = case shown="True" w350 {
              tunnel: w368 -> [w413 w419]
              tunnel: w367 -> [w411 w418]
              tunnel: [w375 w417] -> w365
              tunnel: [w374 w416] -> w364
              frame False {
                n193 = call-poly <vilib>:"KwRL-motion-move-linear.vi"("error in"=w413, "position"=T4 {"X"=134.0, "Y"=-135.0, "Z"=-150.0, "O"=0.0, "A"=0.0, "T"=0.0, "S"=0.0}, "robot session"=w411) -> ("error out"=w410:errorcluster, "robot session*"=w412:string)  [unwired: 7 in]
                n194 = call-poly <vilib>:"KwRL-motion-move-linear.vi"("error in"=w410, "position"=T4 {"X"=85.0, "Y"=380.0, "Z"=-150.0, "O"=90.0, "A"=0.0, "T"=0.0, "S"=0.0}, "robot session"=w412) -> ("error out"=w408:errorcluster, "robot session*"=w407:string)  [unwired: 7 in]
                n195 = call-poly <vilib>:"KwRL-motion-move-linear.vi"("error in"=w408, "position"=T4 {"X"=85.0, "Y"=380.0, "Z"=-240.0, "O"=90.0, "A"=0.0, "T"=0.0, "S"=0.0}, "robot session"=w407) -> ("error out"=w394:errorcluster, "robot session*"=w395:string)  [unwired: 7 in]
                n196 = call <vilib>:"KwRL-in_out-hand-hand_action.vi"("error in"=w394, "value"=TRUE, "clamp"=i16 1, "robot session"=w395) -> ("error out"=w405:errorcluster, "robot session*"=w406:string)  [unwired: 6 in]
                n197 = call <vilib>:"KwRL-in_out-hand-hand_action.vi"("error in"=w405, "value"=TRUE, "clamp"=i16 2, "robot session"=w406) -> ("error out"=w396:errorcluster, "robot session*"=w401:string)  [unwired: 6 in]
                n198 = call-poly <vilib>:"KwRL-motion-move-linear.vi"("error in"=w396, "position"=T4 {"X"=85.0, "Y"=380.0, "Z"=-240.0, "O"=90.0, "A"=0.0, "T"=0.0, "S"=0.0}, "robot session"=w401) -> ("error out"=w393:errorcluster, "robot session*"=w397:string)  [unwired: 7 in]
                n199 = call-poly <vilib>:"KwRL-motion-move-linear.vi"("error in"=w393, "position"=T4 {"X"=85.0, "Y"=380.0, "Z"=-150.0, "O"=90.0, "A"=0.0, "T"=0.0, "S"=0.0}, "robot session"=w397) -> ("error out"=w391:errorcluster, "robot session*"=w390:string)  [unwired: 7 in]
                n200 = call-poly <vilib>:"KwRL-motion-move-linear.vi"("error in"=w391, "position"=T4 {"X"=134.0, "Y"=148.0, "Z"=-150.0, "O"=0.0, "A"=0.0, "T"=0.0, "S"=0.0}, "robot session"=w390) -> ("error out"=w387:errorcluster, "robot session*"=w388:string)  [unwired: 7 in]
                n201 = call-poly <vilib>:"KwRL-motion-move-linear.vi"("error in"=w387, "position"=T4 {"X"=134.0, "Y"=148.0, "Z"=-270.0, "O"=0.0, "A"=0.0, "T"=0.0, "S"=0.0}, "robot session"=w388) -> ("error out"=w379:errorcluster, "robot session*"=w380:string)  [unwired: 7 in]
                n202 = call <vilib>:"KwRL-in_out-hand-hand_action.vi"("error in"=w379, "value"=FALSE, "clamp"=i16 1, "robot session"=w380) -> ("error out"=w384:errorcluster, "robot session*"=w383:string)  [unwired: 6 in]
                n203 = call <vilib>:"KwRL-in_out-hand-hand_action.vi"("error in"=w384, "value"=FALSE, "clamp"=i16 2, "robot session"=w383) -> ("error out"=w376:errorcluster, "robot session*"=w377:string)  [unwired: 6 in]
                n204 = call-poly <vilib>:"KwRL-motion-move-linear.vi"("error in"=w376, "position"=T4 {"X"=134.0, "Y"=148.0, "Z"=-200.0, "O"=0.0, "A"=0.0, "T"=0.0, "S"=0.0}, "robot session"=w377) -> ("error out"=w374:errorcluster, "robot session*"=w375:string)  [unwired: 7 in]
              }
              frame True {
                n205 = call-poly <vilib>:"KwRL-motion-move-linear.vi"("error in"=w419, "position"=T4 {"X"=0.0, "Y"=0.0, "Z"=0.0, "O"=0.0, "A"=0.0, "T"=0.0, "S"=0.0}, "robot session"=w418) -> ("error out"=w416:errorcluster, "robot session*"=w417:string)  [unwired: 7 in]
              }
            }
            n206 = local read "Fahr"() -> (w363:bool)
            n207 = Select(t=T5."deckel", s=w350, f=T5."grundkorper") -> (s? t:f=w354:T5)
            n208 = Select(t=w354, s=w363, f=T5."Bereit") -> (s? t:f=w359:T5)
            n209 = local read "STOP"() -> (w361:bool)
            n210 = Select(t=T5."ende", s=w361, f=w359) -> (s? t:f=w358:T5)
          }
          frame "bolzen" {
            n211 = local write "Schleichfahrt"(FALSE ("Schleichfahrt")) -> ()
            n212 = local write "Rucksetzen"(TRUE ("Rucksetzen")) -> ()
            n213 = local write "LF"(FALSE ("LF")) -> ()
            n214 = local write "RF"(FALSE ("RF")) -> ()
            n215 = local read "HALT"() -> (w424:bool)
            n216 = local read "Fahr"() -> (w426:bool)
            n217 = local read "WIEDERANFAHRT"() -> (w425:bool)
            n218 = Or(x=w425, y=w426) -> (x .or. y?=w427:bool)
            n219 = And(x=w424, y=w427) -> (x .and. y?=w421:bool)
            n220 = case shown="False" w421 {
              tunnel: w442 -> [w453 w486]
              tunnel: w441 -> [w452 w485]
              tunnel: [w446 w483] -> w436
              tunnel: [w445 w484] -> w435
              frame False {
                n221 = local write "Zylinder Bolzen"(TRUE ("Rucksetzen")) -> ()
                n222 = local write "Zylinder Festhalten"(TRUE ("Rucksetzen")) -> ()
                n223 = call-poly <vilib>:"KwRL-motion-move-linear.vi"("error in"=w452, "position"=T4 {"X"=85.0, "Y"=380.0, "Z"=-150.0, "O"=90.0, "A"=0.0, "T"=0.0, "S"=0.0}, "robot session"=w453) -> ("error out"=w455:errorcluster, "robot session*"=w456:string)  [unwired: 7 in]
                n224 = call-poly <vilib>:"KwRL-motion-move-linear.vi"("error in"=w455, "position"=T4 {"X"=155.0, "Y"=380.0, "Z"=-255.0, "O"=0.0, "A"=0.0, "T"=0.0, "S"=0.0}, "robot session"=w456) -> ("error out"=w467:errorcluster, "robot session*"=w468:string)  [unwired: 7 in]
                n225 = call <vilib>:"KwRL-in_out-hand-hand_action.vi"("error in"=w467, "value"=TRUE, "clamp"=i16 1, "robot session"=w468) -> ("error out"=w471:errorcluster, "robot session*"=w472:string)  [unwired: 6 in]
                n226 = call <vilib>:"KwRL-in_out-hand-hand_action.vi"("error in"=w471, "value"=TRUE, "clamp"=i16 2, "robot session"=w472) -> ("error out"=w458:errorcluster, "robot session*"=w464:string)  [unwired: 6 in]
                n227 = call-poly <vilib>:"KwRL-motion-move-linear.vi"("error in"=w458, "position"=T4 {"X"=155.0, "Y"=380.0, "Z"=-255.0, "O"=0.0, "A"=0.0, "T"=0.0, "S"=0.0}, "robot session"=w464) -> ("error out"=w454:errorcluster, "robot session*"=w451:string)  [unwired: 7 in]
                n228 = call-poly <vilib>:"KwRL-motion-move-linear.vi"("error in"=w454, "position"=T4 {"X"=155.0, "Y"=380.0, "Z"=-150.0, "O"=0.0, "A"=0.0, "T"=0.0, "S"=0.0}, "robot session"=w451) -> ("error out"=w459:errorcluster, "robot session*"=w460:string)  [unwired: 7 in]
                n229 = call-poly <vilib>:"KwRL-motion-move-linear.vi"("error in"=w459, "position"=T4 {"X"=155.0, "Y"=-135.0, "Z"=-150.0, "O"=0.0, "A"=0.0, "T"=0.0, "S"=0.0}, "robot session"=w460) -> ("error out"=w450:errorcluster, "robot session*"=w449:string)  [unwired: 7 in]
                n230 = call-poly <vilib>:"KwRL-motion-move-linear.vi"("error in"=w450, "position"=T4 {"X"=134.0, "Y"=-135.0, "Z"=-270.0, "O"=0.0, "A"=0.0, "T"=0.0, "S"=0.0}, "robot session"=w449) -> ("error out"=w447:errorcluster, "robot session*"=w448:string)  [unwired: 7 in]
                n231 = call <vilib>:"KwRL-in_out-hand-hand_action.vi"("error in"=w447, "value"=FALSE, "clamp"=i16 1, "robot session"=w448) -> ("error out"=w477:errorcluster, "robot session*"=w476:string)  [unwired: 6 in]
                n232 = call <vilib>:"KwRL-in_out-hand-hand_action.vi"("error in"=w477, "value"=FALSE, "clamp"=i16 2, "robot session"=w476) -> ("error out"=w446:errorcluster, "robot session*"=w445:string)  [unwired: 6 in]
              }
              frame True {
                n233 = local write "Zylinder Bolzen"(FALSE ("Rucksetzen")) -> ()
                n234 = local write "Zylinder Festhalten"(FALSE ("Rucksetzen")) -> ()
                n235 = call-poly <vilib>:"KwRL-motion-move-linear.vi"("error in"=w485, "position"=T4 {"X"=0.0, "Y"=0.0, "Z"=0.0, "O"=0.0, "A"=0.0, "T"=0.0, "S"=0.0}, "robot session"=w486) -> ("error out"=w483:errorcluster, "robot session*"=w484:string)  [unwired: 7 in]
              }
            }
            n236 = local read "Fahr"() -> (w434:bool)
            n237 = Select(t=T5."bolzen", s=w421, f=T5."deckel") -> (s? t:f=w428:T5)
            n238 = Select(t=w428, s=w434, f=T5."Bereit") -> (s? t:f=w430:T5)
            n239 = local read "STOP"() -> (w432:bool)
            n240 = Select(t=T5."ende", s=w432, f=w430) -> (s? t:f=w429:T5)
          }
          frame "grundkorper" {
            n241 = local write "Zylinder Bolzen"(FALSE ("Rucksetzen")) -> ()
            n242 = local write "Schleichfahrt"(FALSE ("Schleichfahrt")) -> ()
            n243 = local write "Zylinder Festhalten"(FALSE ("Rucksetzen")) -> ()
            n244 = local write "Rucksetzen"(TRUE ("Rucksetzen")) -> ()
            n245 = local write "LF"(FALSE ("LF")) -> ()
            n246 = local write "RF"(FALSE ("RF")) -> ()
            n247 = local read "HALT"() -> (w492:bool)
            n248 = local read "Fahr"() -> (w494:bool)
            n249 = local read "WIEDERANFAHRT"() -> (w493:bool)
            n250 = Or(x=w493, y=w494) -> (x .or. y?=w495:bool)
            n251 = And(x=w492, y=w495) -> (x .and. y?=w488:bool)
            n252 = case shown="False" w488 {
              tunnel: w505 -> [w526 w556]
              tunnel: w504 -> [w525 w557]
              tunnel: [w523 w554] -> w503
              tunnel: [w522 w555] -> w502
              frame False {
                n253 = call-poly <vilib>:"KwRL-motion-move-linear.vi"("error in"=w526, "position"=T4 {"X"=134.0, "Y"=148.0, "Z"=-150.0, "O"=0.0, "A"=0.0, "T"=0.0, "S"=0.0}, "robot session"=w525) -> ("error out"=w528:errorcluster, "robot session*"=w529:string)  [unwired: 7 in]
                n254 = call-poly <vilib>:"KwRL-motion-move-linear.vi"("error in"=w528, "position"=T4 {"X"=85.0, "Y"=380.0, "Z"=-150.0, "O"=90.0, "A"=0.0, "T"=0.0, "S"=0.0}, "robot session"=w529) -> ("error out"=w519:errorcluster, "robot session*"=w520:string)  [unwired: 7 in]
                n255 = call-poly <vilib>:"KwRL-motion-move-linear.vi"("error in"=w519, "position"=T4 {"X"=85.0, "Y"=380.0, "Z"=-280.0, "O"=90.0, "A"=0.0, "T"=0.0, "S"=0.0}, "robot session"=w520) -> ("error out"=w518:errorcluster, "robot session*"=w517:string)  [unwired: 7 in]
                n256 = call <vilib>:"KwRL-in_out-hand-hand_action.vi"("error in"=w518, "value"=TRUE, "clamp"=i16 1, "robot session"=w517) -> ("error out"=w524:errorcluster, "robot session*"=w543:string)  [unwired: 6 in]
                n257 = call <vilib>:"KwRL-in_out-hand-hand_action.vi"("error in"=w524, "value"=TRUE, "clamp"=i16 2, "robot session"=w543) -> ("error out"=w531:errorcluster, "robot session*"=w538:string)  [unwired: 6 in]
                n258 = call-poly <vilib>:"KwRL-motion-move-linear.vi"("error in"=w531, "position"=T4 {"X"=85.0, "Y"=380.0, "Z"=-280.0, "O"=90.0, "A"=0.0, "T"=0.0, "S"=0.0}, "robot session"=w538) -> ("error out"=w527:errorcluster, "robot session*"=w534:string)  [unwired: 7 in]
                n259 = call-poly <vilib>:"KwRL-motion-move-linear.vi"("error in"=w527, "position"=T4 {"X"=85.0, "Y"=380.0, "Z"=-150.0, "O"=90.0, "A"=0.0, "T"=0.0, "S"=0.0}, "robot session"=w534) -> ("error out"=w532:errorcluster, "robot session*"=w533:string)  [unwired: 7 in]
                n260 = call-poly <vilib>:"KwRL-motion-move-linear.vi"("error in"=w532, "position"=T4 {"X"=134.0, "Y"=-70.0, "Z"=-150.0, "O"=0.0, "A"=0.0, "T"=0.0, "S"=0.0}, "robot session"=w533) -> ("error out"=w514:errorcluster, "robot session*"=w515:string)  [unwired: 7 in]
                n261 = call-poly <vilib>:"KwRL-motion-move-linear.vi"("error in"=w514, "position"=T4 {"X"=134.0, "Y"=-70.0, "Z"=-270.0, "O"=0.0, "A"=0.0, "T"=0.0, "S"=0.0}, "robot session"=w515) -> ("error out"=w513:errorcluster, "robot session*"=w512:string)  [unwired: 7 in]
                n262 = call <vilib>:"KwRL-in_out-hand-hand_action.vi"("error in"=w513, "value"=FALSE, "clamp"=i16 1, "robot session"=w512) -> ("error out"=w550:errorcluster, "robot session*"=w549:string)  [unwired: 6 in]
                n263 = call <vilib>:"KwRL-in_out-hand-hand_action.vi"("error in"=w550, "value"=FALSE, "clamp"=i16 2, "robot session"=w549) -> ("error out"=w545:errorcluster, "robot session*"=w544:string)  [unwired: 6 in]
                n264 = call-poly <vilib>:"KwRL-motion-move-linear.vi"("error in"=w545, "position"=T4 {"X"=0.0, "Y"=0.0, "Z"=0.0, "O"=0.0, "A"=0.0, "T"=0.0, "S"=0.0}, "robot session"=w544) -> ("error out"=w523:errorcluster, "robot session*"=w522:string)  [unwired: 7 in]
              }
              frame True {
                n265 = call-poly <vilib>:"KwRL-motion-move-linear.vi"("error in"=w556, "position"=T4 {"X"=0.0, "Y"=0.0, "Z"=0.0, "O"=0.0, "A"=0.0, "T"=0.0, "S"=0.0}, "robot session"=w557) -> ("error out"=w554:errorcluster, "robot session*"=w555:string)  [unwired: 7 in]
              }
            }
            n266 = local read "Fahr"() -> (w501:bool)
            n267 = Select(t=T5."grundkorper", s=w488, f=T5."rechtsfahrt2") -> (s? t:f=w491:T5)
            n268 = Select(t=w491, s=w501, f=T5."Bereit") -> (s? t:f=w497:T5)
            n269 = local read "STOP"() -> (w499:bool)
            n270 = Select(t=T5."ende", s=w499, f=w497) -> (s? t:f=w496:T5)
          }
          frame "rechtsfahrt2" {
            n271 = local read "HALT"() -> (w560:bool)
            n272 = local read "Fahr"() -> (w562:bool)
            n273 = local read "WIEDERANFAHRT"() -> (w561:bool)
            n274 = Or(x=w561, y=w562) -> (x .or. y?=w563:bool)
            n275 = And(x=w560, y=w563) -> (x .and. y?=w559:bool)
            n276 = local read "RA"() -> (w573:bool)
            n277 = local read "Fahr"() -> (w570:bool)
            n278 = Select(t=T5."ende", s=w573, f=T5."rechtsfahrt2") -> (s? t:f=w568:T5)
            n279 = case shown="False" w559 {
              frame False {
                n280 = local write "Zylinder Bolzen"(FALSE ("Rucksetzen")) -> ()
                n281 = local write "Zylinder Festhalten"(FALSE ("Rucksetzen")) -> ()
                n282 = local write "Schleichfahrt"(FALSE ("Schleichfahrt")) -> ()
                n283 = local write "Rucksetzen"(TRUE ("Rucksetzen")) -> ()
                n284 = local write "RF"(TRUE ("RF")) -> ()
                n285 = local write "LF"(FALSE ("LF")) -> ()
              }
              frame True {
                n286 = local write "Zylinder Bolzen"(FALSE ("Rucksetzen")) -> ()
                n287 = local write "Zylinder Festhalten"(FALSE ("Rucksetzen")) -> ()
                n288 = local write "Schleichfahrt"(FALSE ("Schleichfahrt")) -> ()
                n289 = local write "Rucksetzen"(TRUE ("Rucksetzen")) -> ()
                n290 = local write "RF"(FALSE ("RF")) -> ()
                n291 = local write "LF"(FALSE ("LF")) -> ()
              }
            }
            n292 = Select(t=w568, s=w570, f=T5."Bereit") -> (s? t:f=w565:T5)
            n293 = local read "STOP"() -> (w567:bool)
            n294 = Select(t=T5."ende", s=w567, f=w565) -> (s? t:f=w564:T5)
          }
          frame "ende" {
            n295 = local write "Zylinder Bolzen"(FALSE ("Rucksetzen")) -> ()
            n296 = local write "Zylinder Festhalten"(FALSE ("Rucksetzen")) -> ()
            n297 = local write "Schleichfahrt"(FALSE ("Schleichfahrt")) -> ()
            n298 = local write "Rucksetzen"(FALSE ("Rucksetzen")) -> ()
            n299 = local write "RF"(FALSE ("RF")) -> ()
            n300 = local write "LF"(FALSE ("LF")) -> ()
            n301 = call-poly <vilib>:"KwRL-motion-move-linear.vi"("error in"=w607, "position"="position 2", "robot session"=w604) -> ("error out"=w603:errorcluster, "robot session*"=w602:string)  [unwired: 7 in]
            n302 = call <vilib>:"KwRL-in_out-hand-hand_action.vi"("error in"=w603, "value"="value", "clamp"=i16 1, "robot session"=w602) -> ("error out"=w596:errorcluster, "robot session*"=w599:string)  [unwired: 6 in]
            n303 = call <vilib>:"KwRL-in_out-hand-hand_action.vi"("error in"=w596, "value"="value 2", "clamp"=i16 2, "robot session"=w599) -> ("error out"=w595:errorcluster, "robot session*"=w594:string)  [unwired: 6 in]
          }
        }
        n304 = call <vilib>:"Simple Error Handler.vi"("error in (no error)"=w74) -> ("error?"=w70:bool, "error out"=w72:errorcluster)  [unwired: 4 in, 3 out]
      }
    }
    n305 = global read "cRIO_FPGA_COMMUNICATION Global.vi" "Stop"() -> (w58:bool)
    n306 = Or(x=w57, y=w58) -> (x .or. y?=w56:bool)
  }
  n307 = call <vilib>:"KwRL-close_session.vi"("error in"=w2, "robot session"=w5) -> ()  [unwired: 8 in, 2 out]
